vi "获取最新一笔数据.vi"(8 "错误输入（无错误）":errorcluster, 10 "ping":bool, 11 "table":string) -> (0 "错误输出":errorcluster, 2 "检测值":cluster{"时间":timestamp, "检测值":dbl}, 3 "data":dbl)   [LabVIEW 2016]
uses:
  <vilib>/addons/database/Connection.llb/DB Tools Open Connec (String).vi
  <vilib>/addons/database/Connection.llb/Conn Execute.vi
  <vilib>/addons/database/Recordset.llb/Rec Fetch Recordset Data (R).vi
  <vilib>/addons/database/Recordset.llb/Rec Destroy - Connection.vi
  <userlib>/_LVST/sqlite_api/Core/Query/SQLite_Query-Standard.vi
  <vilib>/addons/database/_DB Variant To Data/Database Variant To Data.xnode
  <vilib>/addons/database/NI_Database_API.lvlib
  SQLite/SQLite Lib.lvlib
  Access/Access Lib.lvlib
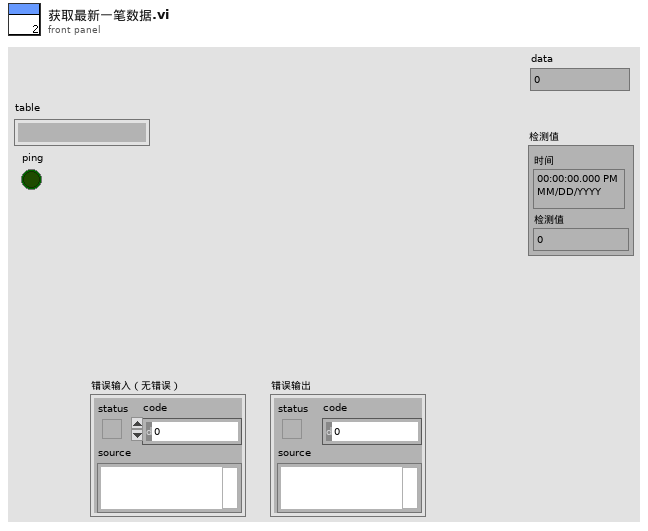
[diagram p1: front panel]
types:
  T1 = typedef "数据库类型.ctl" = enum16{"Access", "SQLite"}
  T2 = typedef "NI_Database_API.lvlib/Conn ObjectReference.ctl" = refnum<k1>
  T3 = typedef "NI_Database_API.lvlib/Rec ObjectReference.ctl" = refnum<k1>
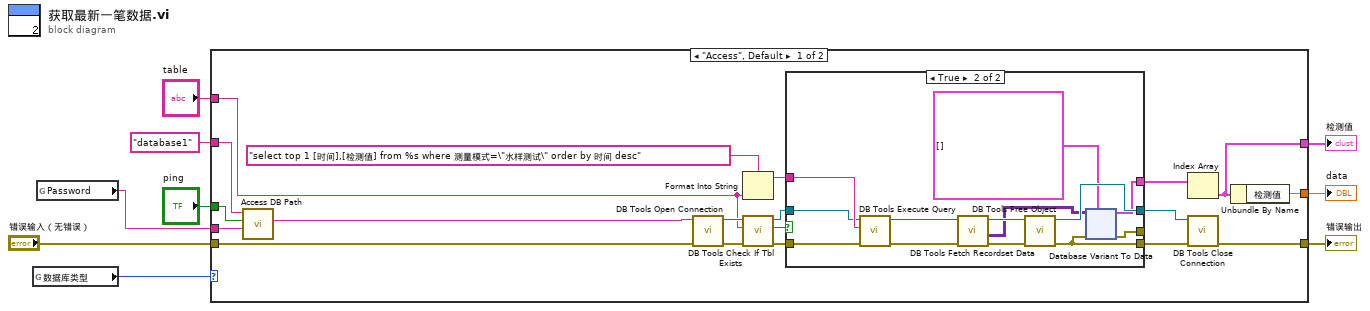
[diagram p0: block diagram]
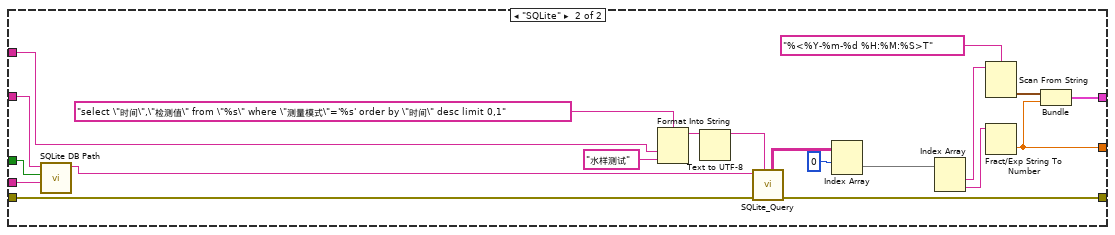
[diagram p3: hidden frame]
diagram:
  n1 = global read "外部调用接口全局变量.vi" "数据库类型"() -> (w2:T1)
  n2 = global read "外部调用接口全局变量.vi" "Password"() -> (w1:string)
  n3 = case shown="\"Access\", Default" w2 {
    tunnel: "table" -> [w13 w145]
    tunnel: [w21 w139] -> w8
    tunnel: "错误输入（无错误）" -> [w25 w142]
    tunnel: [w10 w143] -> w6
    tunnel: "database1" ("database") -> [w24 w147]
    tunnel: [w22 w137] -> w4
    tunnel: "ping" -> [w20 w132]
    tunnel: w1 -> [w18 w129]
    frame "Access", Default {
      n4 = call "Access DB Path.vi"("Password"=w18, "ping"=w20, "database"=w24) -> ("Connection information"=w19:string)  [unwired: 7 in, 1 out]
      n5 = call-poly <vilib>:"DB Tools Open Connection.vi"("error in (no error)"=w25, "connection information"=w19) -> ("error out"=w15:errorcluster, "connection reference"=w17:T2)  [unwired: 6 in]
      n6 = Format Into String(format string="select top 1 [时间],[检测值] from %s where 测量模式=\"水样测试\" order by 时间 desc" ("格式字符串"), w13) -> (resulting string=w26:string)  [unwired: 2 in, 1 out]
      n7 = call <vilib>:"DB Tools Check If Tbl Exists.vi"("error in (no error)"=w15, "table name"=w13, "connection reference"=w17) -> ("error out"=w14:errorcluster, "exists?"=w12:bool, "connection reference out"=w16:T2)  [unwired: 2 out]
      n8 = case shown="True" w12 {
        tunnel: [w30 w39] -> w27
        tunnel: [w29 w31] -> w11
        tunnel: w26 -> [_ w38]
        tunnel: [_ w37] -> _
        tunnel: [_ w34] -> w23
        tunnel: w16 -> [w30 w33]
        tunnel: w14 -> [w29 w32]
        frame False {
        }
        frame True {
          n9 = call-poly <vilib>:"DB Tools Execute Query.vi"("error in (no error)"=w32, "SQL query"=w38, "connection reference"=w33) -> ("error out"=w40:errorcluster, "recordset reference"=w43:T3)  [unwired: 5 in]
          n10 = call-poly <vilib>:"DB Tools Fetch Recordset Data.vi"("error in (no error)"=w40, "recordset reference"=w43) -> ("error out"=w41:errorcluster, "recordset data"=w35:variant[][], "recordset reference out"=w42:T3)  [unwired: 3 in]
          n11 = call-poly <vilib>:"DB Tools Free Object.vi"("error in (no error)"=w41, "recordset reference"=w42) -> ("error out"=w31:errorcluster, "connection reference"=w39:T2)  [unwired: 8 in]
          n12 = xnode "Database Variant To Data"("database variant"=w35, "error in (no error)"=w31, "type"=cluster{"时间":timestamp, "检测值":dbl}[] []) -> ("data"=w34:cluster{"时间":timestamp, "检测值":dbl}[], "error out"=w37:errorcluster)
        }
      }
      n13 = Index Array(array=w23) -> (element=w22:cluster{"时间":timestamp, "检测值":dbl})  [unwired: 1 in]
      n14 = call <vilib>:"DB Tools Close Connection.vi"("error in (no error)"=w11, "connection reference"=w27) -> ("error out"=w10:errorcluster)  [unwired: 5 in]
      n15 = Unbundle By Name(w22) -> ("检测值"=w21:dbl)
    }
    frame "SQLite" {
      n16 = call "SQLite DB Path.vi"("Password"=w129, "ping"=w132, "database"=w147) -> ("Path out"=w148:string)  [unwired: 8 in]
      n17 = Format Into String(format string="select \"时间\",\"检测值\" from \"%s\" where \"测量模式\"='%s' order by \"时间\" desc limit 0,1" ("格式字符串"), w145, "水样测试" ("String")) -> (resulting string=w135:string)  [unwired: 2 in, 1 out]
      n18 = Text to UTF-8(11:w135) -> (3:w134:string)  [unwired: 2 in, 1 out]
      n19 = call-poly <userlib>:"SQLite_Query.vi"("SQL Query"=w134, "error in (no error)"=w142, "DB Path"=w148) -> ("error out"=w143:errorcluster, "Results"=w133:string[][])  [unwired: 3 in, 2 out]
      n20 = Index Array(array=w133, index (row)=0 ("索引 (行)")) -> (element=w130:string[])  [unwired: 1 in]
      n21 = Index Array(array=w130) -> (element #1=w136:string, element #2=w141:string)  [unwired: 2 in]
      n22 = Scan From String(format string="%<%Y-%m-%d %H:%M:%S>T" ("格式字符串"), input string=w136) -> (output 1=w138:timestamp)  [unwired: 3 in, 3 out]
      n23 = Fract/Exp String To Number(string=w141) -> (number=w139:dbl)  [unwired: 3 in, 1 out]
      n24 = Bundle(w138, w139) -> (w137:cluster{timestamp, dbl})  [unwired: 1 in]
    }
  }
  "错误输出" <- w6
  "data" <- w8
  "检测值" <- w4
